vi "clear_plot_data.vi"(6 "clear all?":bool, 8 "error in (no error)":errorcluster, 10 "PrepLineObjectName":string) -> (0 "error out":errorcluster)   [LabVIEW 2017]
doc: "clears the value-history data of the given \"PrepLineObject\" or of all objects. Of \"clear all\" is selected, there's no need to wire the PreLineObject Name"
uses:
  Classes/PrepLineObject/PrepLineObject.lvclass
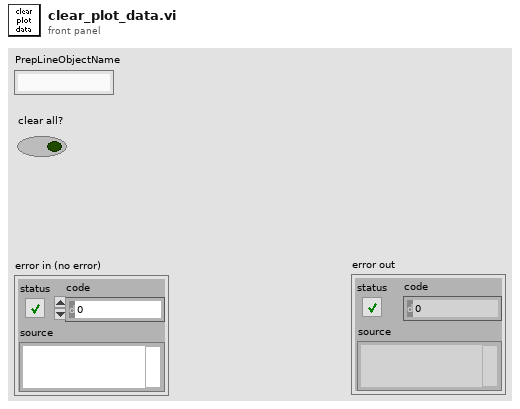
[diagram p1: front panel]
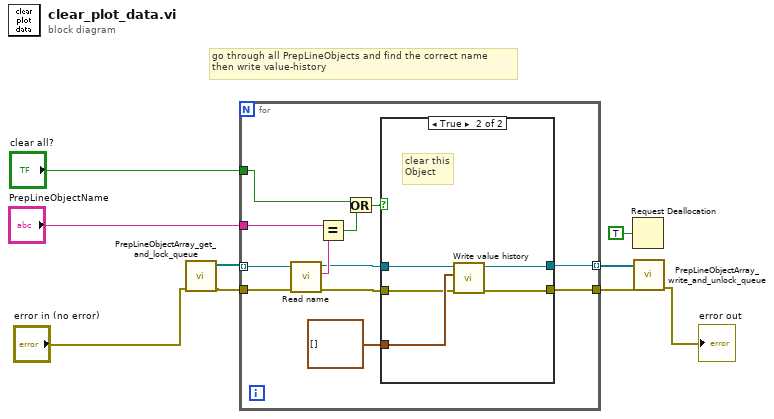
[diagram p0: block diagram]
diagram:
  # "go through all PrepLineObjects and find the correct name\nthen write value-history"
  n1 = call "PrepLineObjectArray_get_and_lock_queue.vi"("error in (no error)"="error in (no error)") -> ("error out"=w4:errorcluster, "PrepLineObjects"=w7:refnum<class "PrepLineObject.lvclass">[])  [unwired: 9 in]
  n2 = for {
    tunnel: w7 -> [w21] mode=indexing
    tunnel: "PrepLineObjectName" -> [w19]
    tunnel: [w15] -> w3
    tunnel: [w16] -> w6 mode=indexing
    tunnel: "clear all?" -> [w12]
    tunnel: w4 -> [w10]
    n3 = call-dynamic "Read name.vi"("error in (no error)"=w10, "PrepLineObject in"=w21) -> ("error out"=w17:errorcluster, "name"=w20:string, "PrepLineObject out"=w18:refnum<class "PrepLineObject.lvclass">)  [unwired: 7 in]
    n4 = Equal?(x=w19, y=w20) -> (x = y?=w13:bool)
    n5 = Or(x=w12, y=w13) -> (x .or. y?=w11:bool)
    n6 = case shown="True" w11 {
      tunnel: w18 -> [w23 w27]
      tunnel: w17 -> [w22 w26]
      tunnel: [w23 w25] -> w16
      tunnel: [w22 w24] -> w15
      tunnel: cluster{"time as number":dbl, "Value":dbl}[] [] ("value history") -> [_ w28]
      frame False {
        # "not the\ncorrect object"
      }
      frame True {
        # "clear this\nObject"
        n7 = call-dynamic "Write value history.vi"("error in (no error)"=w26, "value history"=w28, "PrepLineObject in"=w27) -> ("error out"=w24:errorcluster, "PrepLineObject out"=w25:refnum<class "PrepLineObject.lvclass">)  [unwired: 7 in]
      }
    }
  }
  n8 = Request Deallocation(TRUE ("flag")) -> ()
  n9 = call "PrepLineObjectArray_write_and_unlock_queue.vi"("error in (no error)"=w3, "PrepLineObjArray"=w6) -> ("error out"=→"error out":errorcluster)  [unwired: 9 in]
